vi "SimplexTest_Linear.vi"() -> ()   [LabVIEW 2014]
uses:
  Simplex_Engine_Controls.ctl
  Standard Action.ctl
panel:
  out "x Values - Amount of Modes Out":dbl[][](array[numeric])
  out "F(x) - Evaluation Results Out":dbl[](array[numeric])
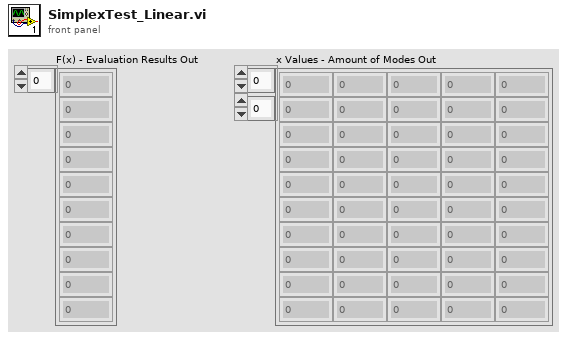
[diagram p1: front panel]
types:
  T1 = typedef "Standard Action.ctl" = enum16{"Read", "Write"}
  T2 = typedef "Simplex_Engine_Controls.ctl" = enum16{"Initialize", "Compute Centroid", "Sort", "Evaluate", "Switch", "Get Reflection", "Get Expansion", "Get Contraction", "Get Reduction", "Exit"}
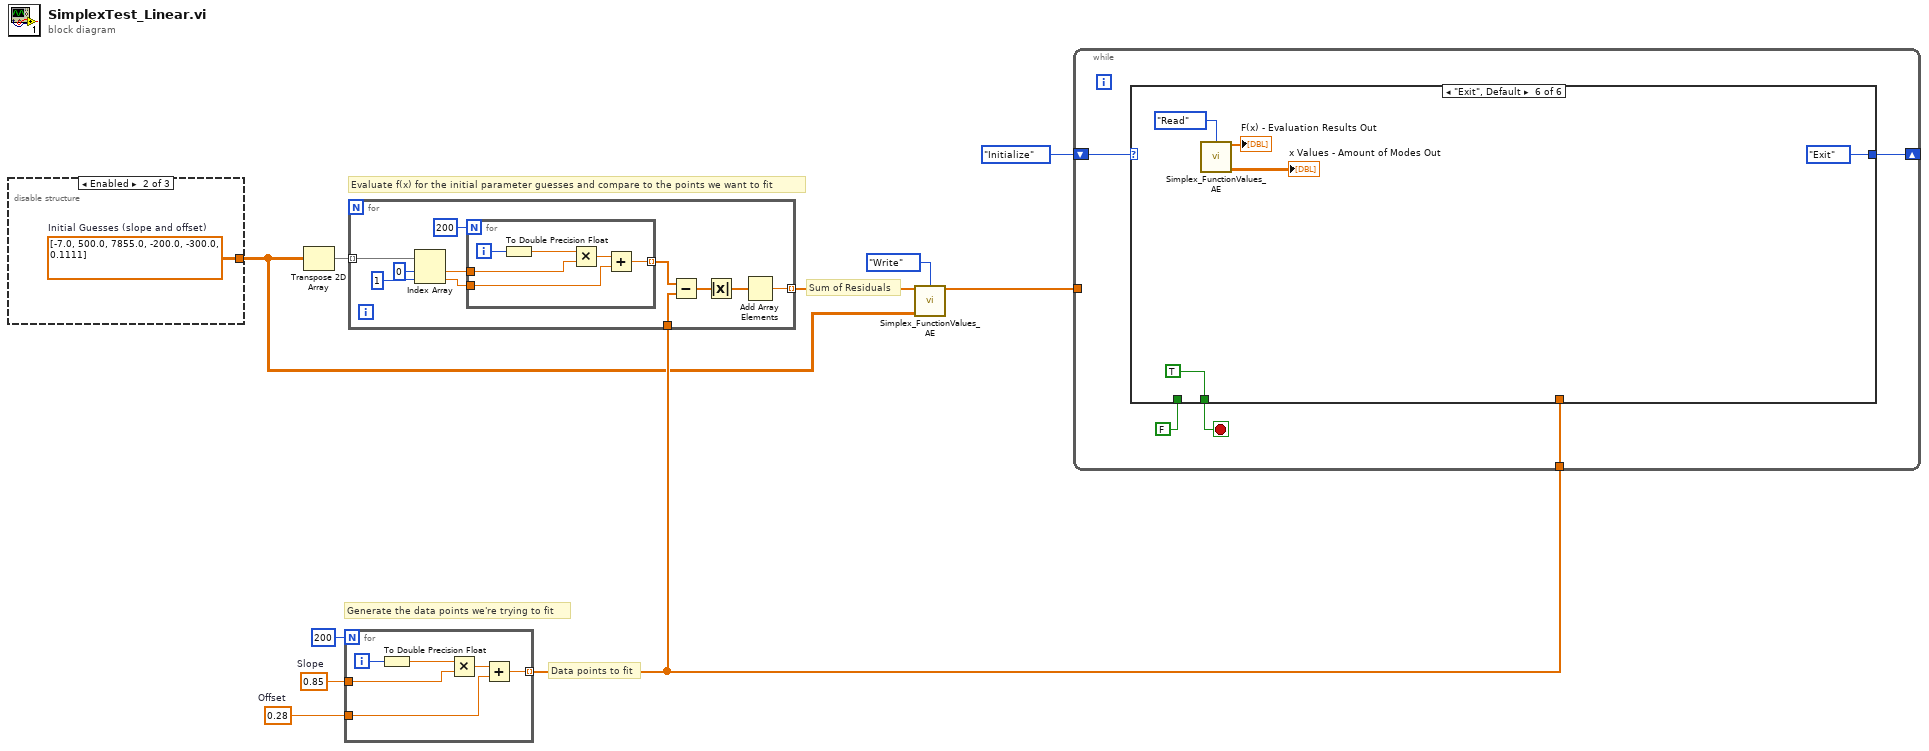
[diagram p0: block diagram]
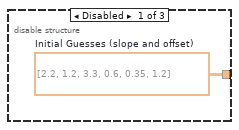
[diagram p2: hidden frame]
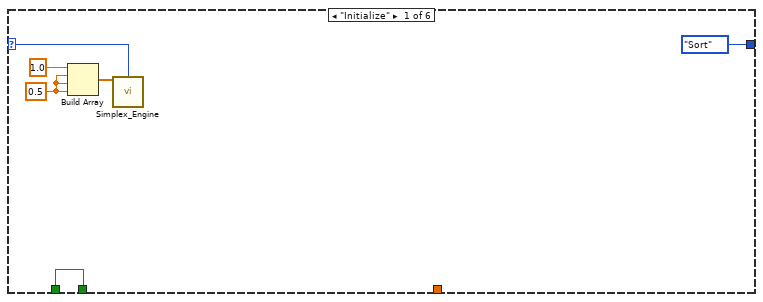
[diagram p4: hidden frame]
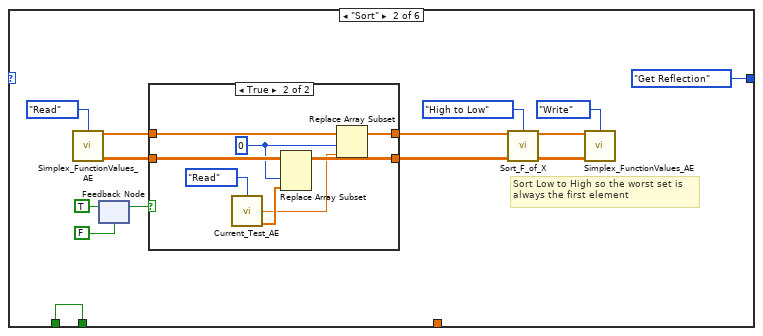
[diagram p5: hidden frame]
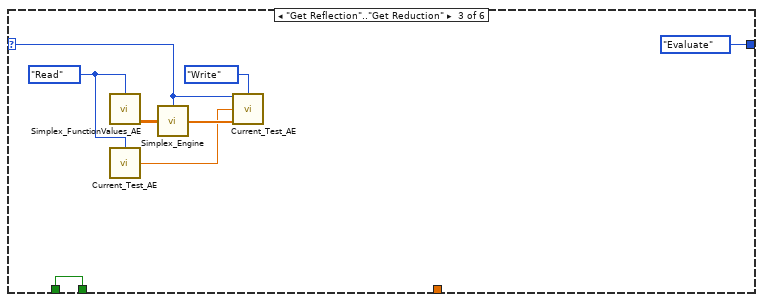
[diagram p7: hidden frame]
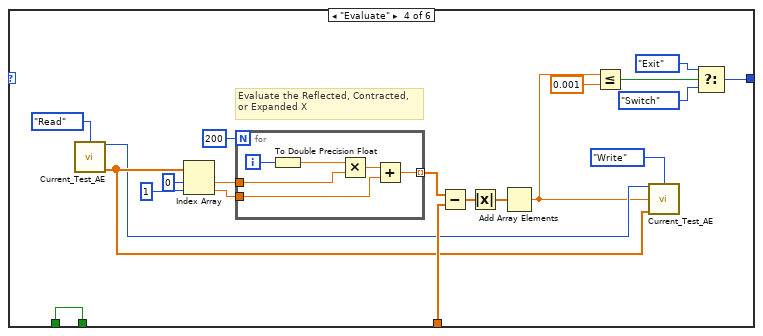
[diagram p8: hidden frame]
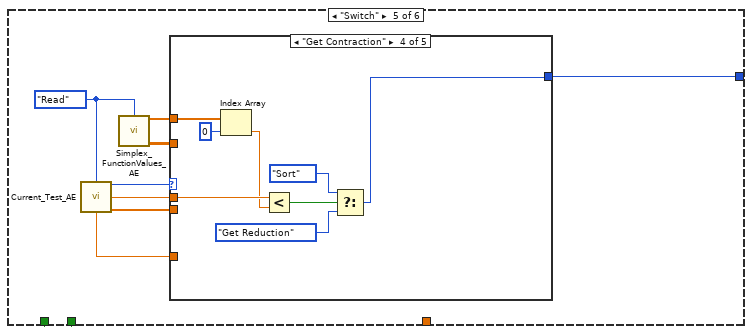
[diagram p9: hidden frame]
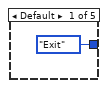
[diagram p10: hidden frame]
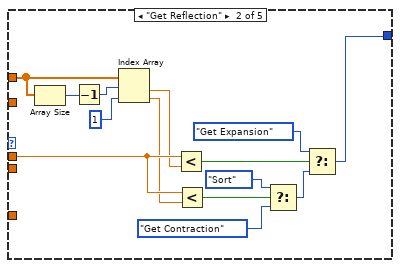
[diagram p11: hidden frame]
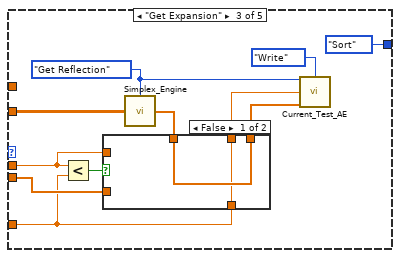
[diagram p12: hidden frame]
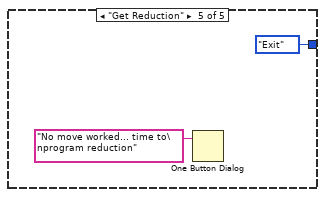
[diagram p14: hidden frame]
diagram:
  w10 = 0.28  # Offset
  w9 = 0.85  # Slope
  # "Sum of Residuals"
  # "Evaluate f(x) for the initial parameter guesses and compare to the points we want to fit"
  # "Data points to fit"
  # "Generate the data points we're trying to fit"
  n1 = disable-structure shown="Enabled" {
    disable-tunnel: [w11 w12 _] -> w2
    frame Disabled {
      w11 = dbl[][] [[2.2, 1.2, 3.3], [0.6, 0.35, 1.2]]  # Initial Guesses (slope and offset)
    }
    frame Enabled {
      w12 = dbl[][] [[-7.0, 500.0, 7855.0], [-200.0, -300.0, 0.1111]]  # Initial Guesses (slope and offset)
    }
    frame Disabled {
    }
  }
  n2 = Transpose 2D Array(2D array=w2) -> (transposed array=w7:dbl[][])
  n3 = for {
    N: 200 -> [_]
    tunnel: [w15] -> w5 mode=indexing
    tunnel: w10 -> [w14]
    tunnel: w9 -> [w13]
    i -> [w18]
    n4 = To Double Precision Float(number=w18) -> (double precision float=w17:dbl)
    n5 = Multiply(x=w17, y=w13) -> (x*y=w16:dbl)
    n6 = Add(x=w16, y=w14) -> (x+y=w15:dbl)
  }
  n7 = for {
    tunnel: w7 -> [w29] mode=indexing
    tunnel: w5 -> [w22]
    tunnel: [w19] -> w3 mode=indexing
    n8 = Index Array(array=w29, index #1=0 ("index"), index #2=1 ("index")) -> (element #1=w25:dbl, element #2=w24:dbl)
    n9 = for {
      N: 200 -> [_]
      tunnel: [w32] -> w23 mode=indexing
      tunnel: w24 -> [w31]
      tunnel: w25 -> [w30]
      i -> [w35]
      n10 = To Double Precision Float(number=w35) -> (double precision float=w34:dbl)
      n11 = Multiply(x=w34, y=w30) -> (x*y=w33:dbl)
      n12 = Add(x=w33, y=w31) -> (x+y=w32:dbl)
    }
    n13 = Subtract(x=w23, y=w22) -> (x-y=w21:dbl[])
    n14 = Absolute Value(x=w21) -> (abs(x)=w20:dbl[])
    n15 = Add Array Elements(numeric array=w20) -> (sum=w19:dbl)
  }
  n16 = call "Simplex_FunctionValues_AE.vi"("F(x) - Evaluation Results"=w3, "Action"=Standard_Action."Write", "x Values - Amount of Modes"=w2) -> ("F(x) - Evaluation Results Out"=w1:dbl[])  [unwired: 11 in, 1 out]
  n17 = while {
    shift-right: [w39] -> _
    shift-left: Simplex_Engine_Controls."Initialize" ("Actions") -> [w40]
    tunnel: w5 -> [w38]
    tunnel: w1 -> [_]
    stop <- w36 stop-if-true
    n18 = case shown="\"Exit\", Default" w40 {
      selector: w40 -> [w41 _ w76 _ _ _]
      tunnel: [Simplex_Engine_Controls."Sort" ("Actions") Simplex_Engine_Controls."Get Reflection" ("Actions") Simplex_Engine_Controls."Evaluate" ("Actions") w81 w109 Simplex_Engine_Controls."Exit" ("Actions")] -> w39
      tunnel: w38 -> [_ _ _ w98 _ _]
      tunnel: FALSE -> [w42 w48 w71 w85 w105 _]
      tunnel: [w42 w48 w71 w85 w105 TRUE] -> w36
      frame "Initialize" {
        w45 = 0.5 ("element")
        n19 = Build Array(1.0, w45, w45, w45) -> (w43:dbl[])
        n20 = call "Simplex_Engine.vi"("Simplex Parameters"=w43, "Actions"=w41) -> ()  [unwired: 13 in, 1 out]
      }
      frame "Sort" {
        # "Sort Low to High so the worst set is\nalways the first element"
        n21 = call "Simplex_FunctionValues_AE.vi"("Action"=Standard_Action."Read") -> ("F(x) - Evaluation Results Out"=w55:dbl[], "x Values - Amount of Modes Out"=w53:dbl[][])  [unwired: 13 in]
        n22 = feedback-in #1(TRUE) -> ()
        n23 = feedback #1(FALSE) -> (w49:bool)
        n24 = case shown="True" w49 {
          tunnel: w55 -> [w62 w70]
          tunnel: [w62 w69] -> w54
          tunnel: w53 -> [w61 w68]
          tunnel: [w61 w67] -> w52
          frame False {
          }
          frame True {
            w65 = 0 ("index")
            n25 = call "Current_Test_AE.vi"("Action"=Standard_Action."Read") -> ("Test F(x) Out"=w63:dbl, "Test X Out"=w64:dbl[])  [unwired: 11 in, 2 out]
            n26 = Replace Array Subset(array=w68, new element=w64, index (col)=w65) -> (w67:dbl[][])  [unwired: 1 in]
            n27 = Replace Array Subset(array=w70, new element=w63, index=w65) -> (w69:dbl[])
          }
        }
        n28 = call "Sort_F_of_X.vi"("F(x) - Evaluation Results"=w54, "Sort Direction"=enum16{"Low to High", "High to Low"}."High to Low", "x Values - Amount of Modes"=w52) -> ("Sorted F(x)"=w60:dbl[], "Sorted X Values"=w59:dbl[][])  [unwired: 11 in]
        n29 = call "Simplex_FunctionValues_AE.vi"("F(x) - Evaluation Results"=w60, "Action"=Standard_Action."Write", "x Values - Amount of Modes"=w59) -> ()  [unwired: 11 in, 2 out]
      }
      frame "Get Reflection".."Get Reduction" {
        w72 = Standard_Action."Read" ("Action")
        n30 = call "Simplex_FunctionValues_AE.vi"("Action"=w72) -> ("x Values - Amount of Modes Out"=w78:dbl[][])  [unwired: 13 in, 1 out]
        n31 = call "Current_Test_AE.vi"("Action"=w72) -> ("Test F(x) Out"=w73:dbl)  [unwired: 11 in, 3 out]
        n32 = call "Simplex_Engine.vi"("Actions"=w76, "x Values - Amount of Modes"=w78) -> ("Test X"=w77:dbl[])  [unwired: 13 in]
        n33 = call "Current_Test_AE.vi"("Current Action"=w76, "Action"=Standard_Action."Write", "Test F(x)"=w73, "Test X"=w77) -> ()  [unwired: 8 in, 4 out]
      }
      frame "Evaluate" {
        # "Evaluate the Reflected, Contracted,\nor Expanded X"
        n34 = call "Current_Test_AE.vi"("Action"=Standard_Action."Read") -> ("Current Action Out"=w86:T2, "Test X Out"=w87:dbl[])  [unwired: 11 in, 2 out]
        n35 = Index Array(array=w87, index #1=0 ("index"), index #2=1 ("index")) -> (element #1=w94:dbl, element #2=w93:dbl)
        n36 = for {
          N: 200 -> [_]
          tunnel: [w101] -> w92 mode=indexing
          tunnel: w93 -> [w100]
          tunnel: w94 -> [w99]
          i -> [w104]
          n37 = To Double Precision Float(number=w104) -> (double precision float=w103:dbl)
          n38 = Multiply(x=w103, y=w99) -> (x*y=w102:dbl)
          n39 = Add(x=w102, y=w100) -> (x+y=w101:dbl)
        }
        n40 = Subtract(x=w92, y=w98) -> (x-y=w91:dbl[])
        n41 = Absolute Value(x=w91) -> (abs(x)=w90:dbl[])
        n42 = Add Array Elements(numeric array=w90) -> (sum=w84:dbl)
        n43 = Less Or Equal?(x=w84, y=0.001) -> (x <= y?=w83:bool)
        n44 = call "Current_Test_AE.vi"("Current Action"=w86, "Action"=Standard_Action."Write", "Test F(x)"=w84, "Test X"=w87) -> ()  [unwired: 8 in, 4 out]
        n45 = Select(t=Simplex_Engine_Controls."Exit", s=w83, f=Simplex_Engine_Controls."Switch" ("Actions")) -> (s? t:f=w81:T2)
      }
      frame "Switch" {
        w110 = Standard_Action."Read" ("Action")
        n46 = call "Current_Test_AE.vi"("Action"=w110) -> ("Current Action Out"=w112:T2, "Test F(x) Out"=w111:dbl, "Reflection F(x)"=w106:dbl, "Test X Out"=w107:dbl[])  [unwired: 11 in]
        n47 = call "Simplex_FunctionValues_AE.vi"("Action"=w110) -> ("F(x) - Evaluation Results Out"=w113:dbl[], "x Values - Amount of Modes Out"=w108:dbl[][])  [unwired: 13 in]
        n48 = case shown="\"Get Contraction\"" w112 {
          tunnel: w111 -> [_ w126 w134 w149 _]
          tunnel: w113 -> [_ w127 _ w151 _]
          tunnel: [Simplex_Engine_Controls."Exit" ("f") w115 Simplex_Engine_Controls."Sort" ("f") w144 Simplex_Engine_Controls."Exit" ("f")] -> w109
          tunnel: w108 -> [_ _ w136 _ _]
          tunnel: w107 -> [_ _ w133 _ _]
          tunnel: w106 -> [_ _ w129 _ _]
          frame Default {
          }
          frame "Get Reflection" {
            n49 = Array Size(array=w127) -> (size(s)=w128:i32)
            n50 = Decrement(x=w128) -> (x-1=w123:i32)
            n51 = Index Array(array=w127, index #1=w123, index #2=1 ("index")) -> (element #1=w124:dbl, element #2=w125:dbl)
            n52 = Less?(x=w126, y=w124) -> (x < y?=w120:bool)
            n53 = Less?(x=w126, y=w125) -> (x < y?=w119:bool)
            n54 = Select(t=Simplex_Engine_Controls."Sort" ("Actions"), s=w119, f=Simplex_Engine_Controls."Get Contraction") -> (s? t:f=w118:T2)
            n55 = Select(t=Simplex_Engine_Controls."Get Expansion" ("Actions"), s=w120, f=w118) -> (s? t:f=w115:T2)
          }
          frame "Get Expansion" {
            w138 = Simplex_Engine_Controls."Get Reflection" ("Actions")
            n56 = Less?(x=w134, y=w129) -> (x < y?=w135:bool)
            n57 = call "Simplex_Engine.vi"("Actions"=w138, "x Values - Amount of Modes"=w136) -> ("Test X"=w130:dbl[])  [unwired: 13 in]
            n58 = case shown="False" w135 {
              tunnel: w134 -> [_ w143]
              tunnel: w133 -> [_ w142]
              tunnel: [w140 w143] -> w132
              tunnel: [w141 w142] -> w131
              tunnel: w130 -> [w141 _]
              tunnel: w129 -> [w140 _]
              frame False {
              }
              frame True {
              }
            }
            n59 = call "Current_Test_AE.vi"("Current Action"=w138, "Action"=Standard_Action."Write", "Test F(x)"=w132, "Test X"=w131) -> ()  [unwired: 8 in, 4 out]
          }
          frame "Get Contraction" {
            n60 = Index Array(array=w151, index=0) -> (element=w148:dbl)
            n61 = Less?(x=w149, y=w148) -> (x < y?=w147:bool)
            n62 = Select(t=Simplex_Engine_Controls."Sort" ("Actions"), s=w147, f=Simplex_Engine_Controls."Get Reduction") -> (s? t:f=w144:T2)
          }
          frame "Get Reduction" {
            n63 = One Button Dialog(message="No move worked... time to\nprogram reduction") -> ()  [unwired: 1 in, 1 out]
          }
        }
      }
      frame "Exit", Default {
        n64 = call "Simplex_FunctionValues_AE.vi"("Action"=Standard_Action."Read") -> ("F(x) - Evaluation Results Out"=→"F(x) - Evaluation Results Out":dbl[], "x Values - Amount of Modes Out"=→"x Values - Amount of Modes Out":dbl[][])  [unwired: 13 in]
      }
    }
  }
